vi "read_calibration_file_v2.vi"(8 "error in (no error)":errorcluster caption="错误输入（无错误）", 9 "通道数量":i32=128, 10 "板子数量":i32=2, 11 "file path (dialog if empty)":path=path "G:/tdc/2017/data/12_codeDensity.csv" caption="文件路径 （空时为对话框）") -> (0 "error out":errorcluster caption="错误输出", 1 "code_density":i64[][](array[numeric]), 2 "accumulation":u32[][](array[numeric]), 3 "Cal Table":u32[](array[numeric])=[100002, 100002, 100002, 100002, 100002, 100002, 100002, 100002, 100002, 100002, 100002, 100002, 100002, 100002, 100002, 100002, 100002, 100002, 100002, 100002, 100002, 100002, 100002, 100002, 100002, 100002, 100002, 100002, 100002, 100002, 100002, 100002, 100002, 100002, 100002, 100002, 100002, 100002, 100002, 100002, 100002, 100002, 100002, 100002, 100002, 100002, 100002, 100002, 100002, 100002, 100002, 100002, 100002, 100002, 100002, 100002, 100002, 100002, 100002, 100002, 100002, 100002, 100002, 100002, 100002, 100002, 100002, 100002, 100002, 100002, 100002, 100002, 100002, 100002, 100002, 100002, 100002, 100002, 100002, 100002, 100002, 100002, 100002, 100002, 100002, 100002, 100002, 100002, 100002, 100002, 100002, 100002, 100002, 100002, 100002, 100002, 100002, 100002, 100002, 100002, 100002, 100002, 100002, 100002, 100002, 100002, 100002, 100002, 100002, 100002, 100002, 100002, 100002, 100002, 100002, 100002, 100002, 100002, 100002, 100002, 100002, 100002, 100002, 100002, 100002, 100002, 100002, 100002])   [LabVIEW 2017]
uses:
  <vilib>/Utility/file.llb/Read Delimited Spreadsheet (I64).vi
panel:
  out "大小 3":i32[](array[numeric])=[2048, 128]
  out "大小 2":i32[](array[numeric])=[2048, 256]
  out "Array":u32[][](array[numeric])
  out "大小":i32[](array[numeric])=[2048, 128]
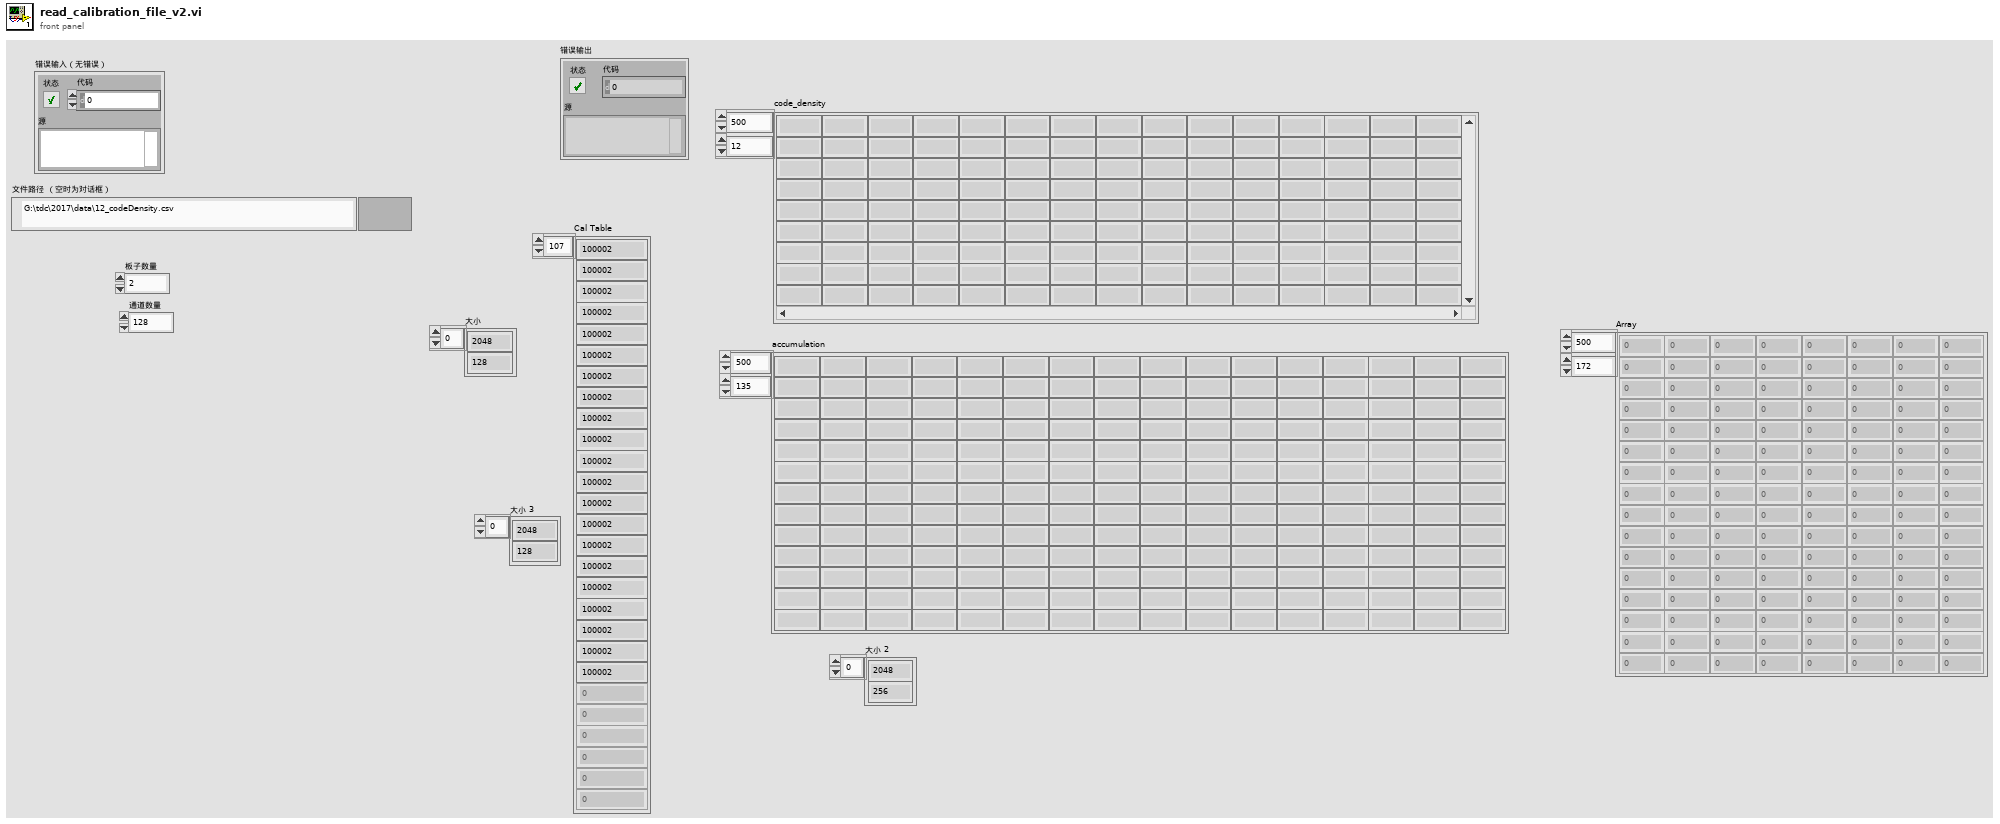
[diagram p1: front panel]
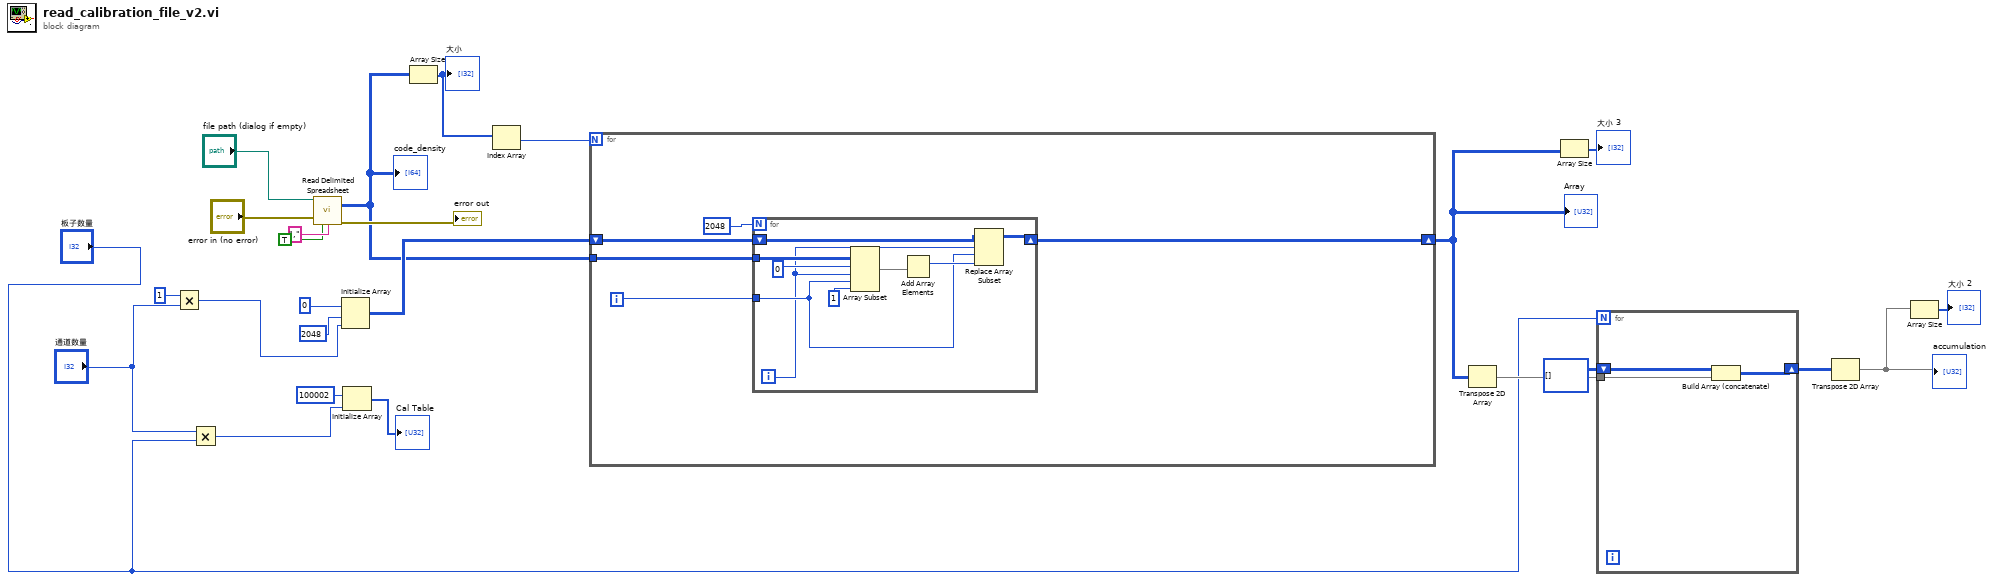
[diagram p0: block diagram]
diagram:
  n1 = Multiply(x=1, y="通道数量") -> (x*y=w21:i32)
  n2 = Multiply(x="通道数量", y="板子数量") -> (x*y=w1:i32)
  n3 = call-poly <vilib>:"Read Delimited Spreadsheet.vi"("file path (dialog if empty)"="file path (dialog if empty)", "error in (no error)"="error in (no error)", "transpose? (F)"=TRUE, "delimiter (\\t)"="," ("delimiter (\\t)")) -> ("all rows"=w15:i64[][], "error out"=→"error out":errorcluster)  [unwired: 6 in, 4 out]
  "code_density" <- w15
  n4 = Initialize Array(u32 0 ("element"), 2048 ("dimension size"), w21) -> (w20:u32[][])
  n5 = Initialize Array(u32 100002 ("element"), w1) -> (→"Cal Table":u32[])
  n6 = Array Size(array=w15) -> (size(s)=w19:i32[])
  "大小" <- w19
  n7 = Index Array(array=w19) -> (element=w18:i32)  [unwired: 1 in]
  n8 = for {
    N: w18 -> [_]
    shift-right: [w27] -> w9
    shift-left: w20 -> [w30]
    tunnel: w15 -> [w29]
    i -> [w26]
    n9 = for {
      N: 2048 -> [_]
      tunnel: w29 -> [w39]
      tunnel: w26 -> [w32]
      shift-right: [w34] -> w27
      shift-left: w30 -> [w35]
      i -> [w31]
      n10 = Array Subset(array=w39, index (row)=0 ("索引"), length (row)=w31, index (col)=w32, length (col)=1 ("长度")) -> (w36:i64[][])
      n11 = Add Array Elements(numeric array=w36) -> (sum=w33:i64)
      n12 = Replace Array Subset(array=w35, new element=w33, index (row)=w31, index (col)=w32) -> (w34:u32[][])
    }
  }
  "Array" <- w9
  n13 = Transpose 2D Array(2D array=w9) -> (transposed array=w7:u32[][])
  n14 = Array Size(array=w9) -> (size(s)=→"大小 3":i32[])
  n15 = for {
    N: "板子数量" -> [_]
    shift-right: [w41] -> w11
    shift-left: u32[][] [] -> [w42]
    tunnel: w7 -> [w40]
    n16 = Build Array (concatenate)(w42, w40) -> (w41:u32[][])
  }
  n17 = Transpose 2D Array(2D array=w11) -> (transposed array=w6:u32[][])
  "accumulation" <- w6
  n18 = Array Size(array=w6) -> (size(s)=→"大小 2":i32[])
